vi "Cont Acq&Graph Voltage-Int Clk-Analog Start.vi"() -> ()   [LabVIEW 2024]
doc: "I. Description:\nThis example demonstrates how to continuously acquire data (Waveform) using the DAQ device's internal clock and an analog slope start trigger.\n\nII. Instructions for Running:\n1. Select the physical channel to correspond to where your signal is input on the DAQ device.\n2. Enter the minimum and maximum voltage ranges.\nNote: For better accuracy try to match the Input Ranges to the expected voltage level of the measured signal.\n3. Set the rate of the acquisition. Also set the Samples to Read control. This will determine how many samples are read each time the while loop iterates. This also determines how many points are plotted on the graph each iteration.\nNote: The rate should be at least twice as fast as the maximum frequency component of the signal being acquired.\n4. Set the source of the Analog Slope Start Trigger. By default this is APFI0.\n5. Set the slope and level of desired analog edge condition.\n\nIII. Block Diagram Steps:\n1. Create an analog input voltage channel.\n2. Set the rate for the sample clock. Additionally, define the sample mode to be continuous.\n3. Define the parameters for an Analog Slope Start Trigger.\n4. Call the Start VI to start the acquisition.\n5. Read the waveform data in a loop until the user hits the stop button or an error occurs.\n6. Call the Clear Task VI to clear the Task.\n7. Use the popup dialog box to display an error if any.\n\nIV. I/O Connections Overview:\nMake sure your signal input terminal matches the Physical Channel I/O control. Also, make sure your analog trigger terminal matches the Trigger Source Control. For further connection information, refer to your hardware reference manual."
uses:
  <vilib>/Utility/error.llb/DialogType.ctl
  <vilib>/DAQmx/read.llb/DAQmx Read (Analog 1D Wfm NChan NSamp).vi
  <vilib>/DAQmx/create/channels.llb/DAQmx Create Channel (AI-Voltage-Basic).vi
  <vilib>/DAQmx/configure/timing.llb/DAQmx Timing (Sample Clock).vi
  <vilib>/DAQmx/miscellaneous.llb/DAQmx Fill In Error Info.vi
  <vilib>/measure/matone.llb/Extract Multiple Tone Information 1 Chan.vi
  <vilib>/measure/NI_MAPro.lvlib
panel:
  in  "timeout":dbl=100.0
  out "multiple tone information":T1(array[cluster])=[{"detected frequency"=4.909496457635433e-05, "detected amplitude"=5.000672294541098, "detected phase (deg)"=89.47308587110548}, {"detected frequency"=5.499969626560334, "detected amplitude"=0.05006658003932163, "detected phase (deg)"=50.57798674584135}] {"detected phase (deg)" format="%_6g"; "detected amplitude" format="%_6p"; "detected frequency" format="%_6p"}
  in  "Samples to Read":i32=10000
  in  "Physical Channel":tag="cDAQ2Mod7/ai0"
  in  "Minimum Value":dbl=-10.0 format="%0.2f"
  in  "Maximum Value":dbl=10.0 format="%0.2f"
  in  "stop":bool
  in  "Rate":dbl=1000.0 format="%0.2f"
  out "Measurement":waveform(dbl)[](graph)=[{"t0"=timestamp(3368022578.064414 s since 1904-01-01), "dt"=0.00062, "Y"=array[100000 elements], "attributes"=variant("NI_ChannelName"=variant(string "cDAQ2Mod7/ai0"), "NI_UnitDescription"=variant(string "Volts"))}]
  # "For instructions, select Help>>Show Context Help"
  # "Channel Parameters"
  # "Timing Parameters"
  # "*  APFI0 is the default Analog Trigger pin for M Series devices.  \nPlease refer to your device documentation for information \nregarding valid Analog Triggers for your device."
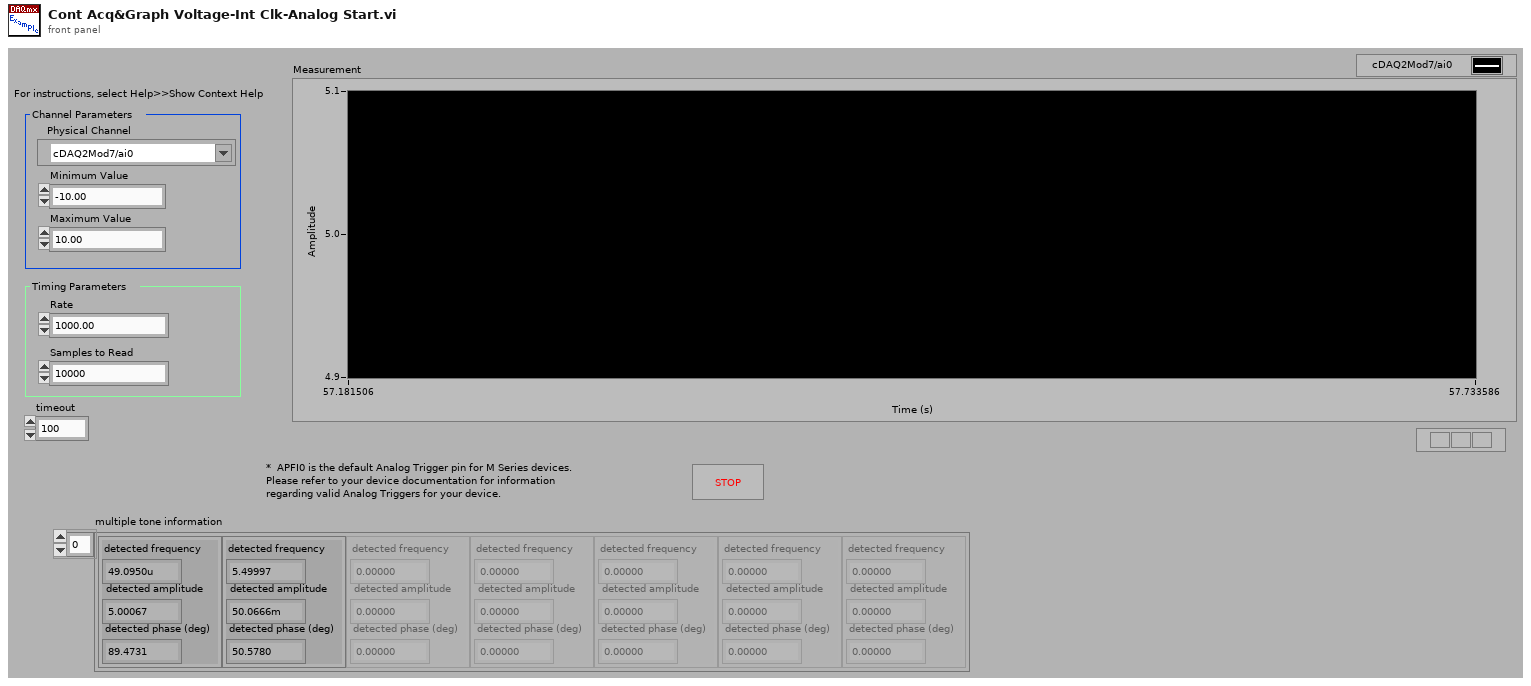
[diagram p1: front panel]
types:
  T1 = cluster{"detected frequency":dbl, "detected amplitude":dbl, "detected phase (deg)":dbl}[]
  T2 = typedef "DialogType.ctl" = u16
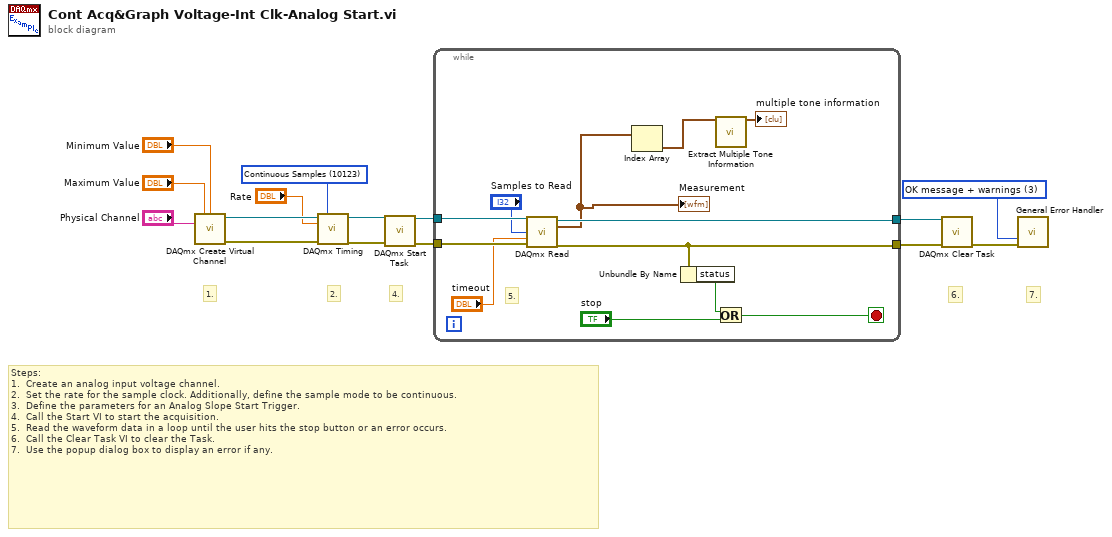
[diagram p0: block diagram]
diagram:
  w1 = T2 3 items=["no dialog", "OK message", "continue or stop message", "OK message + warnings", "continue/stop + warnings"] ("type of dialog (OK msg:1)")
  w6 = 10123 items=["Finite Samples"=10178, "Continuous Samples"=10123] ("sample mode")
  # "7."
  # "6."
  # "Steps: \n1.  Create an analog input voltage channel.\n2.  Set the rate for the sample clock. Additionally, define the sample mode to be continuous.\n3.  Define the parameters for an Analog Slope Start Trigger.\n4.  Call the Start VI to start the acquisition.\n5.  Read the waveform data in a loop until the user hits the stop button or an error occurs.\n6.  Call the Clear Task VI to clear the Task.\n7.  Use the popup dialog box to display an error if any."
  # "4."
  # "2."
  # "1."
  n1 = call-poly <vilib>:"DAQmx Create Virtual Channel.vi"("maximum value"="Maximum Value", "minimum value"="Minimum Value", "physical channels"="Physical Channel") -> ("task out"=w10:refnum<k21>, "error out"=w13:errorcluster)  [unwired: 11 in]
  n2 = call-poly <vilib>:"DAQmx Timing.vi"("task/channels in"=w10, "sample mode"=w6, "rate"="Rate", "error in"=w13) -> ("task out"=w3:refnum<k21>, "error out"=w2:errorcluster)  [unwired: 10 in]
  n3 = call <vilib>:"DAQmx Start Task.vi"("task/channels in"=w3, "error in"=w2) -> ("task out"=w9:refnum<k21>, "error out"=w12:errorcluster)  [unwired: 12 in]
  n4 = while {
    tunnel: w12 -> [w27]
    tunnel: w9 -> [w26]
    tunnel: [w25] -> w8
    tunnel: [w24] -> w5
    stop <- w22 stop-if-true
    # "5."
    n5 = call-poly <vilib>:"DAQmx Read.vi"("task/channels in"=w26, "number of samples per channel"="Samples to Read", "timeout"="timeout", "error in"=w27) -> ("task out"=w25:refnum<k21>, "data"=w18:waveform(dbl)[], "error out"=w24:errorcluster)  [unwired: 9 in]
    "Measurement" <- w18
    n6 = Index Array(array=w18) -> (element=w17:waveform(dbl))  [unwired: 1 in]
    n7 = Unbundle By Name(w24) -> ("status"=w23:bool)
    n8 = call-poly <vilib>:"Extract Multiple Tone Information.vi"("time signal in"=w17) -> ("multiple tone information"=→"multiple tone information":T1)  [unwired: 12 in, 2 out]
    n9 = Or(x=w23, y="stop") -> (x .or. y?=w22:bool)
  }
  n10 = call <vilib>:"DAQmx Clear Task.vi"("task in"=w8, "error in"=w5) -> ("error out"=w11:errorcluster)  [unwired: 13 in]
  n11 = call <vilib>:"General Error Handler.vi"("type of dialog (OK msg:1)"=w1, "error in (no error)"=w11) -> ()  [unwired: 9 in, 5 out]
